vi "Demag_fields.vi"(8 "error in (no error)":errorcluster, 10 "Steps":i32, 11 "Field (T)":dbl format="%.2f") -> (0 "error out":errorcluster, 1 "Fields":dbl[](array[numeric]))   [LabVIEW 2017]
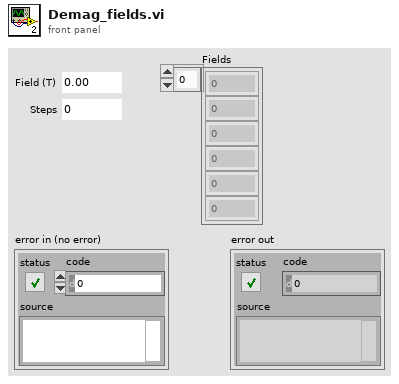
[diagram p1: front panel]
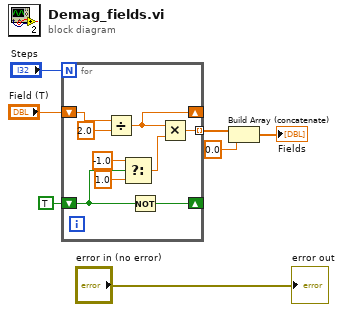
[diagram p0: block diagram]
diagram:
  n1 = for {
    N: "Steps" -> [_]
    shift-right: [w9] -> _
    shift-left: "Field (T)" -> [w16]
    tunnel: [w8] -> w6 mode=indexing
    shift-right: [w14] -> _
    shift-left: TRUE -> [w13]
    n2 = Divide(x=w16, y=2.0) -> (x/y=w9:dbl)
    n3 = Select(t=-1.0 ("y"), s=w13, f=1.0) -> (s? t:f=w10:dbl)
    n4 = Not(x=w13) -> (.not. x?=w14:bool)
    n5 = Multiply(x=w9, y=w10) -> (x*y=w8:dbl)
  }
  n6 = Build Array (concatenate)(w6, 0.0) -> (→"Fields":dbl[])
  "error out" <- "error in (no error)"
